vi "midi_in.disconnect.vi"(8 "error in (no error)":errorcluster, 11 "LabVIEW-MIDI-XPLAT in":refnum<class "LabVIEW-MIDI-XPLAT.lvclass">) -> (0 "error out":errorcluster, 3 "LabVIEW-MIDI-XPLAT out":refnum<class "LabVIEW-MIDI-XPLAT.lvclass">)   [LabVIEW 2020, in "LabVIEW-MIDI-XPLAT.lvclass"]
uses:
  LabVIEW-MIDI-XPLAT.lvclass
  LabVIEW-MIDI-XPLAT.lvclass/LabVIEW-MIDI-XPLAT.ctl
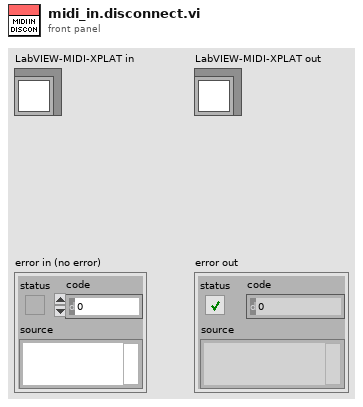
[diagram p1: front panel]
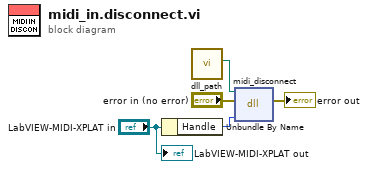
[diagram p0: block diagram]
diagram:
  n1 = Unbundle By Name("LabVIEW-MIDI-XPLAT in") -> ("Handle"=w3:i32)
  n2 = call "dll_path.vi"() -> ("dll"=w4:path)  [unwired: 11 in]
  n3 = dll-call lib="C:/code/LabVIEW-MIDI-XPLAT/dist/TomMIDIllan_*.*" fn="midi_disconnect"(path in=w4, error in="error in (no error)", "handle"=w3) -> (error out=→"error out":errorcluster)  [unwired: 3 in, 1 out]
  "LabVIEW-MIDI-XPLAT out" <- "LabVIEW-MIDI-XPLAT in"
